vi "NewEnchantedMazeGame.vi"(8 "error in (no error)":errorcluster) -> (0 "error out":errorcluster, 3 "EnchantedMazeGame":refnum<class "EnchantedMazeGame.lvclass">)   [LabVIEW 2020, in "FactoryMethod.lvlib" / "NoParametrizedFactoryMethod.lvlib" / "EnchantedMazeGame.lvclass"]
uses:
  EnchantedMazeGame.lvclass
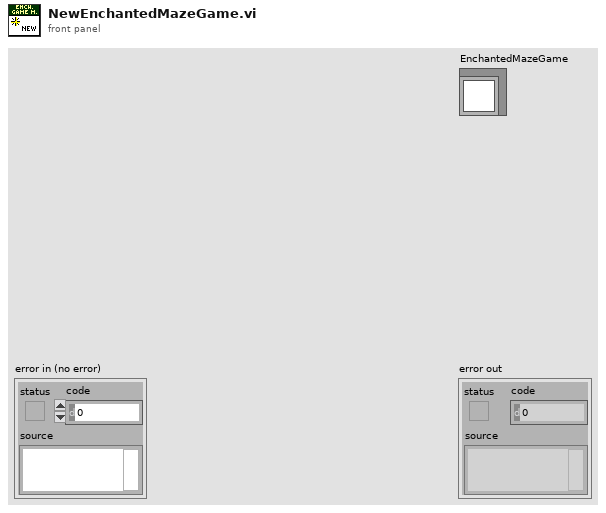
[diagram p1: front panel]
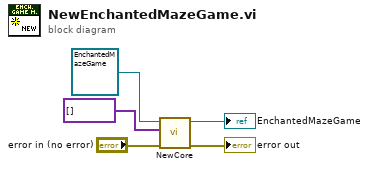
[diagram p0: block diagram]
diagram:
  n1 = call-dynamic "NewCore.vi"("error in (no error)"="error in (no error)", "ParamsArray"=variant[] [], "EnchantedMazeGame"=refnum<class "EnchantedMazeGame.lvclass"> refnum ("ByRef")) -> ("error out"=→"error out":errorcluster, "EnchantedMazeGame"=→"EnchantedMazeGame":refnum<class "EnchantedMazeGame.lvclass">)  [unwired: 7 in]
